vi "Measurement UI.vi"() -> ()   [LabVIEW 2025, in "Example Plugin UI.lvlib"]
uses:
  Example Plugin UI.lvlib
  <vilib>/gRPC/LabVIEW gRPC Library/Shared/grpcId.ctl
  OOB gRPC Client/RPC Messages/hwval_BoolRequest.ctl
  OOB gRPC Client/RPC Messages/hwval_GenericRequest.ctl
  OOB gRPC Client/RPC Messages/hwval_ExportRequest.ctl
  <vilib>/gRPC/LabVIEW gRPC Library/grpc-lvsupport-release.lvlib
  OOB gRPC Client/OOB gRPC Client.lvlib
panel:
  out "Double (Loopback)":dbl
  out "String (Loopback)":string
  in  "Send String":bool
  in  "String":string
  in  "Double":dbl
  in  "Send Double":bool
  in  "Export File Type":string(combo)="RAW"
  out "Status":string
  out "Measurement Logic Counter":i32
  out "OOB gRPC Port":i32
  out "Config String (Loopback)":string
  out "Config Number (Loopback)":dbl
  in  "Config String":string="Text"
  in  "Config Number":dbl=1.0
  in  "Export":bool
  in  "PauseResume":bool caption="Pause"
  out "Export (Loopback)":string
  out "PauseResume (Loopback)":bool
  # "Configuration"
  # "Results"
  # "Interactive"
  # "(These controls are not part of the Measurement Confiugration, This way IS doesn't disable and grey them out)"
  # "Status"
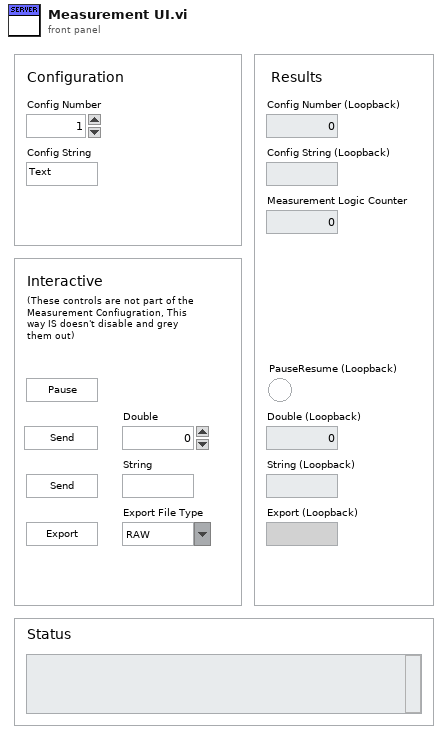
[diagram p1: front panel]
types:
  T1 = typedef "grpc-lvsupport-release.lvlib/grpcId.ctl" = u64
  T2 = typedef "OOB gRPC Client.lvlib/hwval_BoolRequest.ctl" = cluster{"BooleanData":bool}
  T3 = typedef "OOB gRPC Client.lvlib/hwval_GenericRequest.ctl" = cluster{"Command":string, "Payload":u8[]}
  T4 = typedef "OOB gRPC Client.lvlib/hwval_ExportRequest.ctl" = cluster{"FileType":string}
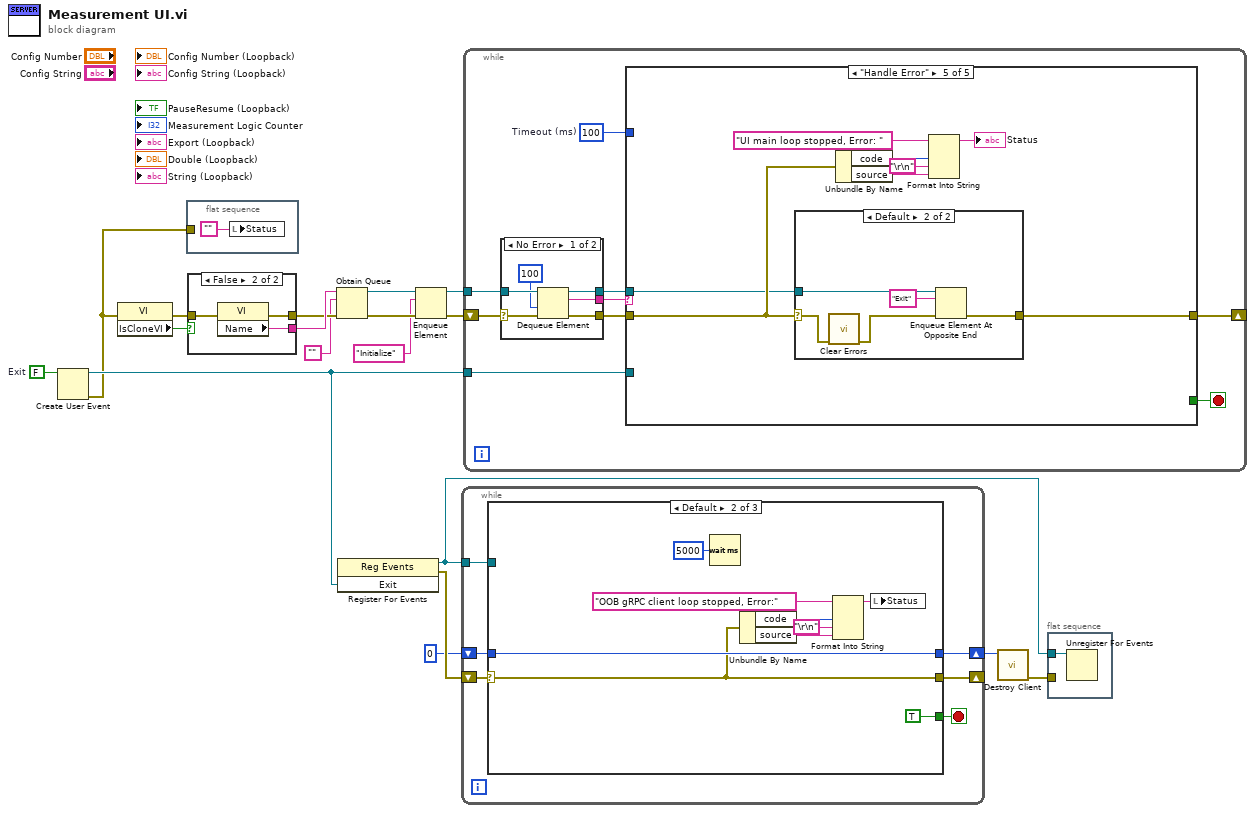
[diagram p0: block diagram]
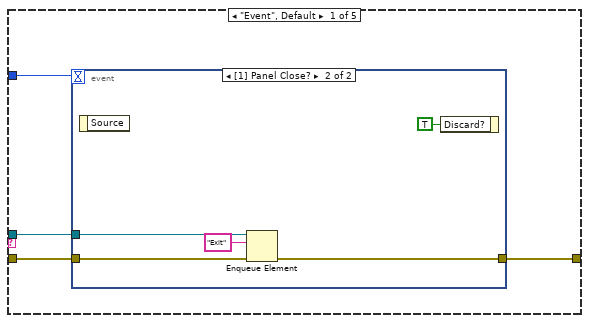
[diagram p2: hidden frame]
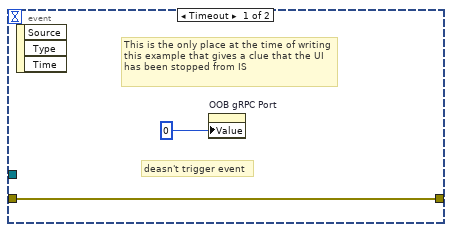
[diagram p3: hidden frame]
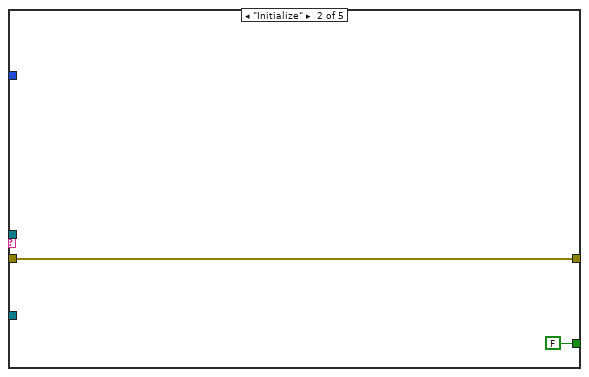
[diagram p4: hidden frame]
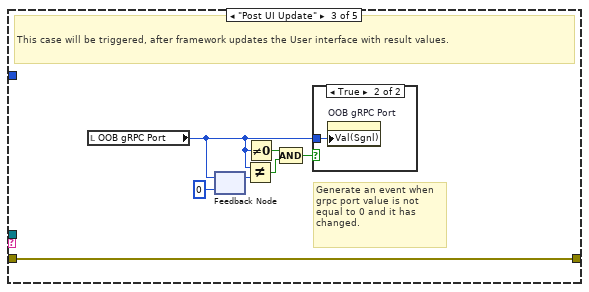
[diagram p5: hidden frame]
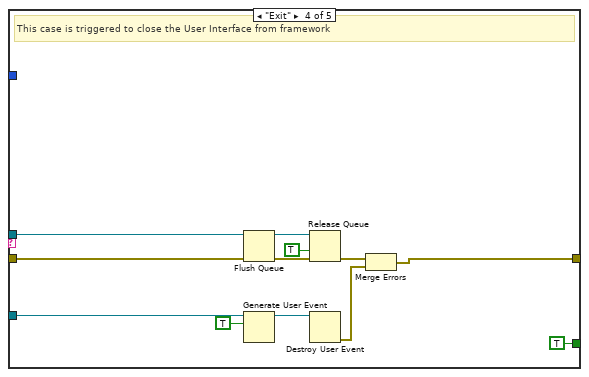
[diagram p7: hidden frame]
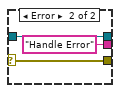
[diagram p9: hidden frame]
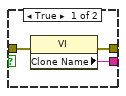
[diagram p10: hidden frame]
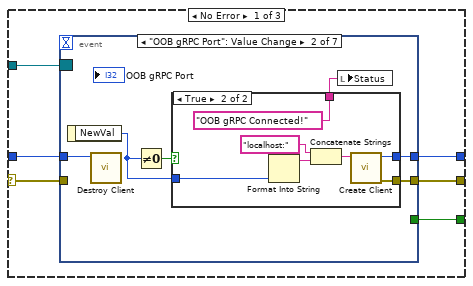
[diagram p11: hidden frame]
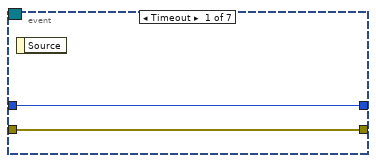
[diagram p12: hidden frame]
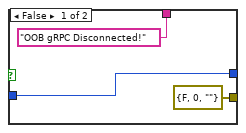
[diagram p13: hidden frame]
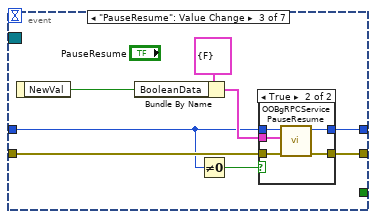
[diagram p14: hidden frame]
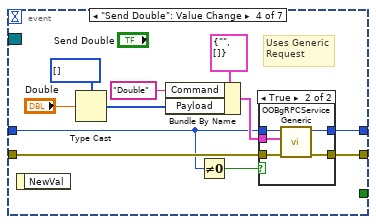
[diagram p16: hidden frame]
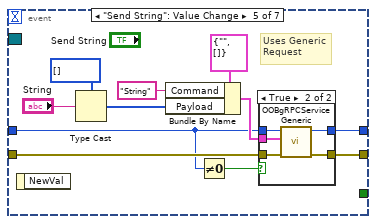
[diagram p18: hidden frame]
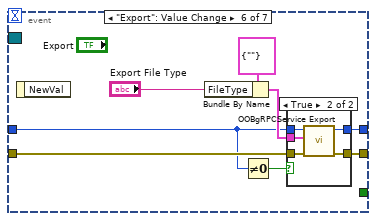
[diagram p20: hidden frame]
diagram:
  w4 = FALSE  # Exit
  n1 = Create User Event(user event datatype=w4) -> (user event=w3:refnum<user-event>, error out=w2:errorcluster)  [unwired: 1 in]
  n2 = property class="VI"(error in=w2) -> (error out=w9:errorcluster, "IsCloneVI"=w14:bool)  [unwired: 1 in, 1 out]
  n3 = flat-sequence {
    tunnel: w2 -> [_]
    frame #0 {
      n4 = local write "Status"("") -> ()
    }
  }
  n5 = case shown="False" w14 {
    tunnel: [w22 w25] -> w13
    tunnel: [w21 w24] -> w18
    tunnel: w9 -> [w20 w23]
    frame True {
      n6 = property class="VI"(error in=w20) -> (error out=w22:errorcluster, "Clone Name"=w21:string)  [unwired: 1 in, 1 out]
    }
    frame False {
      n7 = property class="VI"(error in=w23) -> (error out=w25:errorcluster, "Name"=w24:string)  [unwired: 1 in, 1 out]
    }
  }
  n8 = Obtain Queue(name (unnamed)=w18, element data type="", error in (no error)=w13) -> (queue out=w15:refnum<queue>, error out=w17:errorcluster)  [unwired: 2 in, 1 out]
  n9 = register-events(w3) -> (reference out=w8:refnum<event-registration>, error out=w7:errorcluster)  [unwired: 2 in]
  n10 = Enqueue Element(queue=w15, element="Initialize", error in (no error)=w17) -> (queue out=w10:refnum<queue>, error out=w16:errorcluster)  [unwired: 1 in, 1 out]
  n11 = while {
    tunnel: w8 -> [w28]
    shift-right: [w29] -> _
    shift-left: w7 -> [w31]
    shift-right: [w26] -> w5
    shift-left: T1 0 ("gRPC ID out") -> [w27]
    stop <- w30 stop-if-true
    n12 = case shown="Default" w31 {
      selector: w31 -> [w35 w126 _]
      tunnel: [w32 TRUE w138] -> w30
      tunnel: [w36 w126 errorcluster {"status"=FALSE, "code"=0, "source"=""} ("error IO")] -> w29
      tunnel: w28 -> [w37 _ _]
      tunnel: w27 -> [w34 w132 w135]
      tunnel: [w33 w132 w135] -> w26
      frame No Error {
        n13 = event shown="[1] \"OOB gRPC Port\": Value Change" {
          selector: w37 -> [_ _ _ _ _ _ _]
          dyn-events: _ -> [_ _ _ _ _ _ _]
          timeout: _ -> [_ _ _ _ _ _ _]
          tunnel: [w39 w45 w62 w80 w98 w113 w122] -> w36
          tunnel: w35 -> [w39 _ w61 w79 w97 w112 w122]
          tunnel: w34 -> [w38 w44 w56 w75 w93 w108 w123]
          tunnel: [w38 w43 w63 w81 w99 w114 w123] -> w33
          tunnel: [_ _ _ _ _ _ w124] -> w32
          event Timeout {
            n14 = event-data() -> ()  [unwired: 1 in, 1 out]
          }
          event "OOB gRPC Port": Value Change {
            n15 = event-data() -> ("NewVal"=w41:i32)  [unwired: 1 in]
            n16 = call "Destroy Client.vi"("gRPC ID"=w44) -> ()  [unwired: 10 in, 1 out]
            n17 = Not Equal To 0?(x=w41) -> (x != 0?=w42:bool)
            n18 = case shown="True" w42 {
              tunnel: [errorcluster {"status"=FALSE, "code"=0, "source"=""} ("error out") w55] -> w45
              tunnel: w41 -> [w48 w51]
              tunnel: [w48 w50] -> w43
              tunnel: ["OOB gRPC Disconnected!" ("Status") "OOB gRPC Connected!" ("Status")] -> w40
              frame False {
              }
              frame True {
                n19 = Format Into String(w51) -> (resulting string=w54:string)  [unwired: 3 in, 1 out]
                n20 = Concatenate Strings("localhost:" ("string"), w54) -> (w52:string)
                n21 = call "Create Client.vi"("address"=w52) -> ("error out"=w55:errorcluster, "gRPC ID Out"=w50:T1)  [unwired: 9 in]
              }
            }
            n22 = local write "Status"(w40) -> ()
          }
          event "PauseResume": Value Change {
            n23 = event-data() -> ("NewVal"=w58:bool)  [unwired: 1 in]
            n24 = Bundle By Name(cluster=T2 {"BooleanData"=FALSE} ("Request Data"), "BooleanData"=w58) -> (w59:T2)
            n25 = Not Equal To 0?(x=w56) -> (x != 0?=w57:bool)
            n26 = case shown="True" w57 {
              tunnel: [w65 w70] -> w63
              tunnel: [w64 w69] -> w62
              tunnel: w56 -> [w65 w68]
              tunnel: w61 -> [w64 w67]
              tunnel: w59 -> [_ w66]
              frame False {
              }
              frame True {
                n27 = call "OOBgRPCService PauseResume.vi"("error in"=w67, "Request Data"=w66, "gRPC ID"=w68) -> ("error out"=w69:errorcluster, "gRPC ID out"=w70:T1)  [unwired: 6 in, 1 out]
              }
            }
          }
          event "Send Double": Value Change {
            # "Uses Generic\nRequest"
            n28 = event-data() -> ()  [unwired: 1 in, 1 out]
            n29 = Type Cast(type=u8[] [] ("Payload"), x="Double") -> (*(type *) &x=w71:u8[])
            n30 = Bundle By Name(cluster=T3 {"Command"="", "Payload"=[]} ("Request Data"), "Command"="Double", "Payload"=w71) -> (w77:T3)
            n31 = Not Equal To 0?(x=w75) -> (x != 0?=w76:bool)
            n32 = case shown="True" w76 {
              tunnel: [w83 w88] -> w81
              tunnel: [w82 w87] -> w80
              tunnel: w75 -> [w83 w86]
              tunnel: w79 -> [w82 w85]
              tunnel: w77 -> [_ w84]
              frame False {
              }
              frame True {
                n33 = call "OOBgRPCService Generic.vi"("error in"=w85, "Request Data"=w84, "gRPC ID"=w86) -> ("error out"=w87:errorcluster, "gRPC ID out"=w88:T1)  [unwired: 6 in, 1 out]
              }
            }
          }
          event "Send String": Value Change {
            # "Uses Generic\nRequest"
            n34 = event-data() -> ()  [unwired: 1 in, 1 out]
            n35 = Type Cast(type=u8[] [] ("Payload"), x="String") -> (*(type *) &x=w90:u8[])
            n36 = Bundle By Name(cluster=T3 {"Command"="", "Payload"=[]} ("Request Data"), "Command"="String", "Payload"=w90) -> (w95:T3)
            n37 = Not Equal To 0?(x=w93) -> (x != 0?=w94:bool)
            n38 = case shown="True" w94 {
              tunnel: [w101 w106] -> w99
              tunnel: [w100 w105] -> w98
              tunnel: w93 -> [w101 w104]
              tunnel: w97 -> [w100 w103]
              tunnel: w95 -> [_ w102]
              frame False {
              }
              frame True {
                n39 = call "OOBgRPCService Generic.vi"("error in"=w103, "Request Data"=w102, "gRPC ID"=w104) -> ("error out"=w105:errorcluster, "gRPC ID out"=w106:T1)  [unwired: 6 in, 1 out]
              }
            }
          }
          event "Export": Value Change {
            n40 = event-data() -> ()  [unwired: 1 in, 1 out]
            n41 = Bundle By Name(cluster=T4 {"FileType"=""} ("Request Data"), "FileType"="Export File Type") -> (w110:T4)
            n42 = Not Equal To 0?(x=w108) -> (x != 0?=w109:bool)
            n43 = case shown="True" w109 {
              tunnel: [w116 w121] -> w114
              tunnel: [w115 w120] -> w113
              tunnel: w108 -> [w116 w119]
              tunnel: w112 -> [w115 w118]
              tunnel: w110 -> [_ w117]
              frame False {
              }
              frame True {
                n44 = call "OOBgRPCService Export.vi"("error in"=w118, "Request Data"=w117, "gRPC ID"=w119) -> ("error out"=w120:errorcluster, "gRPC ID out"=w121:T1)  [unwired: 6 in, 1 out]
              }
            }
          }
          event User Event {
            n45 = event-data() -> ("Exit"=w124:bool)  [unwired: 1 in]
          }
        }
      }
      frame Default {
        n46 = Wait (ms)(milliseconds to wait=u32 5000) -> ()  [unwired: 1 out]
        n47 = Unbundle By Name(w126) -> ("code"=w131:i32, "source"=w130:string)
        n48 = Format Into String(initial string="OOB gRPC client loop stopped, Error:" ("format string"), w131, "\r\n", w130) -> (resulting string=w127:string)  [unwired: 2 in, 1 out]
        n49 = local write "Status"(w127) -> ()
      }
      frame Error {
        n50 = local read "OOB gRPC Port"() -> (w140:i32)
        n51 = Wait (ms)(milliseconds to wait=u32 2000) -> ()  [unwired: 1 out]
        n52 = Equal?(x=w140, y=-1 ("x")) -> (x = y?=w138:bool)
        n53 = case shown="False" w138 {
          tunnel: w140 -> [w142 _]
          tunnel: ["OOB gRPC Disconnted!\nReconnecting.." ("Status") "OOB gRPC server side Error.\nMeasrement Logic didn't get the gRPC port from OOB server.\nRestart the plugin." ("Status")] -> w137
          frame False {
            # "triggers event"
            n54 = property on="OOB gRPC Port" class="DigNum (strict)"("Val(Sgnl)"=w142) -> ()  [unwired: 2 in, 2 out]
          }
          frame True {
          }
        }
        n55 = local write "Status"(w137) -> ()
      }
    }
  }
  n56 = while {
    shift-right: [w148] -> _
    shift-left: w16 -> [w152]
    tunnel: w10 -> [w146]
    tunnel: w3 -> [w145]
    stop <- w147 stop-if-true
    w144 = 100  # Timeout (ms)
    n57 = case shown="No Error" w152 {
      selector: w152 -> [w205 w206]
      tunnel: [w204 w206] -> w151
      tunnel: w146 -> [w203 w208]
      tunnel: [w202 w208] -> w150
      tunnel: [w201 "Handle Error"] -> w149
      frame No Error {
        n58 = Dequeue Element(queue=w203, timeout in ms (-1)=100 ("Timeout (ms)"), error in (no error)=w205) -> (queue out=w202:refnum<queue>, element=w201:string, error out=w204:errorcluster)  [unwired: 1 out]
      }
      frame Error {
      }
    }
    n59 = case shown="\"Handle Error\"" w149 {
      tunnel: w151 -> [w155 w164 w172 w185 w189]
      tunnel: w150 -> [w154 _ _ w183 w187]
      tunnel: [w156 w164 w172 w178 w188] -> w148
      tunnel: [_ FALSE _ TRUE _] -> w147
      tunnel: w144 -> [w153 _ _ _ _]
      tunnel: w145 -> [_ _ _ w174 _]
      frame "Event", Default {
        n60 = event shown="[1] Panel Close?" {
          selector: _ -> [_ _]
          dyn-events: _ -> [_ _]
          timeout: w153 -> [_ _]
          tunnel: [w158 w161] -> w156
          tunnel: w155 -> [w158 w162]
          tunnel: w154 -> [_ w160]
          event Timeout {
            # "deasn't trigger event"
            # "This is the only place at the time of writing this example that gives a clue that the UI has been stopped from IS"
            n61 = event-data() -> ()  [unwired: 1 in, 3 out]
            n62 = property on="OOB gRPC Port" class="DigNum (strict)"("Value"=0 ("OOB gRPC Port")) -> ()  [unwired: 2 in, 2 out]
          }
          event Panel Close? {
            n63 = event-data() -> ()  [unwired: 1 in, 1 out]
            n64 = Enqueue Element(queue=w160, element="Exit" ("Message"), error in (no error)=w162) -> (error out=w161:errorcluster)  [unwired: 1 in, 2 out]
            n65 = event-data("Discard?"=TRUE) -> ()  [unwired: 1 in, 1 out]
          }
        }
      }
      frame "Initialize" {
      }
      frame "Post UI Update" {
        # "Generate an event when grpc port value is not equal to 0 and it has changed."
        # "This case will be triggered, after framework updates the User interface with result values."
        n66 = local read "OOB gRPC Port"() -> (w167:i32)
        n67 = feedback-in #1(w167) -> ()
        n68 = feedback #1(0 ("OOB gRPC Port")) -> (w166:i32)
        n69 = Not Equal?(x=w167, y=w166) -> (x != y?=w168:bool)
        n70 = Not Equal To 0?(x=w167) -> (x != 0?=w170:bool)
        n71 = Compound Arithmetic op=AND(w170, w168) -> (w169:bool)
        n72 = case shown="True" w169 {
          tunnel: w167 -> [_ w173]
          frame False {
          }
          frame True {
            n73 = property on="OOB gRPC Port" class="DigNum (strict)"("Val(Sgnl)"=w173) -> ()  [unwired: 2 in, 2 out]
          }
        }
      }
      frame "Exit" {
        # "This case is triggered to close the User Interface from framework"
        n74 = Flush Queue(queue=w183, error in (no error)=w185) -> (queue out=w182:refnum<queue>, error out=w181:errorcluster)  [unwired: 1 out]
        n75 = Generate User Event(user event=w174, event data cluster=TRUE ("event data")) -> (user event out=w176:refnum<user-event>)  [unwired: 2 in, 1 out]
        n76 = Release Queue(queue=w182, force destroy? (F)=TRUE, error in (no error)=w181) -> (error out=w180:errorcluster)  [unwired: 2 out]
        n77 = Destroy User Event(user event=w176) -> (error out=w175:errorcluster)  [unwired: 1 in]
        n78 = Merge Errors(w180, w175) -> (w178:errorcluster)
      }
      frame "Handle Error" {
        n79 = case shown="Default" w189 {
          selector: w189 -> [w194 w199]
          tunnel: [w194 w198] -> w188
          tunnel: w187 -> [_ w196]
          frame No Error {
          }
          frame Default {
            n80 = call <vilib>:"Clear Errors.vi"("error in (no error)"=w199) -> ("error out"=w197:errorcluster)  [unwired: 5 in, 1 out]
            n81 = Enqueue Element At Opposite End(queue=w196, element="Exit", error in (no error)=w197) -> (error out=w198:errorcluster)  [unwired: 1 in, 2 out]
          }
        }
        n82 = Unbundle By Name(w189) -> ("code"=w193:i32, "source"=w192:string)
        n83 = Format Into String(initial string="UI main loop stopped, Error: " ("format string"), w193, "\r\n", w192) -> (resulting string=→"Status":string)  [unwired: 2 in, 1 out]
      }
    }
  }
  n84 = call "Destroy Client.vi"("gRPC ID"=w5) -> ("error out"=w6:errorcluster)  [unwired: 10 in]
  n85 = flat-sequence {
    tunnel: w8 -> [w209]
    tunnel: w6 -> [_]
    frame #0 {
      n86 = Unregister For Events(event registration refnum=w209) -> ()  [unwired: 1 in, 1 out]
    }
  }
